vi "Read Bus Monitor Interface.vi"(10 "Datum Name":string, 11 "IBusMonitor":refnum<class "IBusMonitor.lvclass">) -> (2 "Valid Transport":refnum<class "ITransport.lvclass">, 3 "SubscriptionPolicy Type":refnum<class "ISubscriptionPolicy.lvclass">)   [LabVIEW 2020, in "MonitoredMediator.lvlib" / "IBusMonitor.lvclass"]
uses:
  <vilib>/gpm_packages/@cs/mva-core/Source/MonitoredMediator/IBusMonitor/IBusMonitor.lvclass
  <vilib>/gpm_packages/@cs/transport/Source/ITransport/ITransport.lvclass
  <vilib>/gpm_packages/@cs/mva-core/Source/IMediator/ISubscriptionPolicy/ISubscriptionPolicy.lvclass
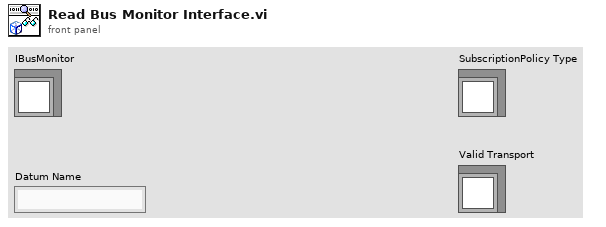
[diagram p1: front panel]
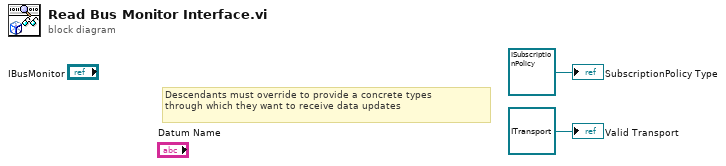
[diagram p0: block diagram]
diagram:
  # "Descendants must override to provide a concrete types\nthrough which they want to receive data updates"
  "Valid Transport" <- refnum<class "ITransport.lvclass"> refnum ("Notification Msg Type")
  "SubscriptionPolicy Type" <- refnum<class "ISubscriptionPolicy.lvclass"> refnum ("Bus Monitor SubscriptionPolicy")
